vi "DIO 1-bit.vi"(8 "DIR":bool, 9 "OUT":bool, 11 "DIO Refnum":refnum<k21>) -> (3 "IN":bool)   [LabVIEW 2015]
doc: "This VI reads a Boolean value from or writes the value to the specified FPGA I/O item according to the direction of the data flow (<b>DIR</b>).\n- DIR: TRUE - Write data to <b>OUT</b>\n- DIR: FALSE - Read data from <b>IN</b>"
uses:
  <vilib>/eio/EIONode/EIONode.xnode
  <vilib>/rvi/eio/common/nirviEmuTemplateMethod_errors.vi
  <vilib>/eio/EIOMethodNode/EIOMethodNode.xnode
panel:
  # "This VI reads a Boolean value from or writes the value to the specified FPGA I/O item according to the direction of the data flow (DIR).\n- DIR: TRUE - Write data to OUT\n- DIR: FALSE - Read data from IN"
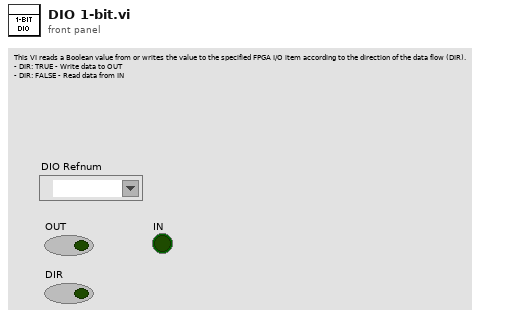
[diagram p1: front panel]
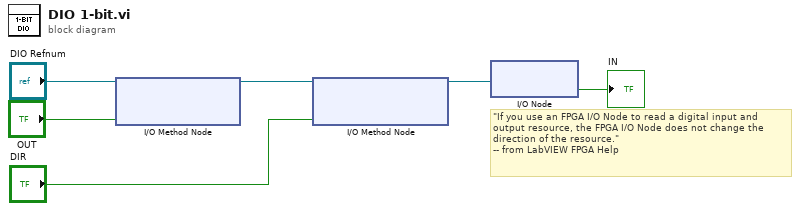
[diagram p0: block diagram]
diagram:
  # "\"If you use an FPGA I/O Node to read a digital input and output resource, the FPGA I/O Node does not change the direction of the resource.\"\n-- from LabVIEW FPGA Help"
  n1 = xnode "I/O Method Node"("FPGA I/O In"="DIO Refnum", "Data"="OUT") -> ("FPGA I/O Out"=w2:refnum<k21>)
  n2 = xnode "I/O Method Node"("FPGA I/O In"=w2, "Enable"="DIR") -> ("FPGA I/O Out"=w1:refnum<k21>)
  n3 = xnode "I/O Node"("FPGA I/O In"=w1) -> ("I/O Item"=→"IN":bool)  [unwired: 1 out]
